vi "ConfigFlattenMicroscopeToXML.vi"(8 "error in (no error)":errorcluster, 11 "MicroscopeArray":string[][](array[string])) -> (0 "error out":errorcluster, 3 "MicrosocopeXML":string)   [LabVIEW 2018, in "Config.lvlib"]
uses:
  Config.lvlib
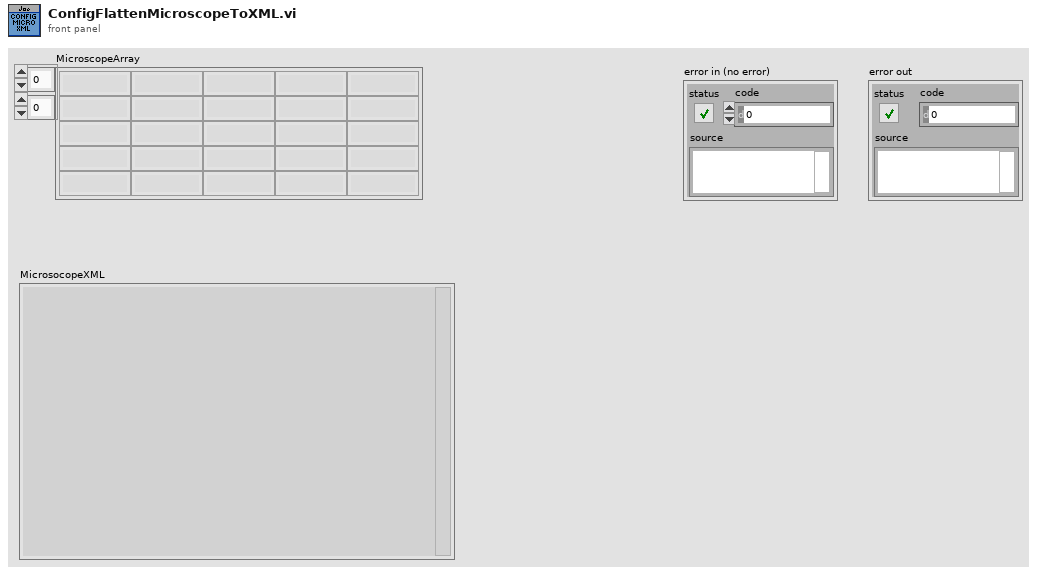
[diagram p1: front panel]
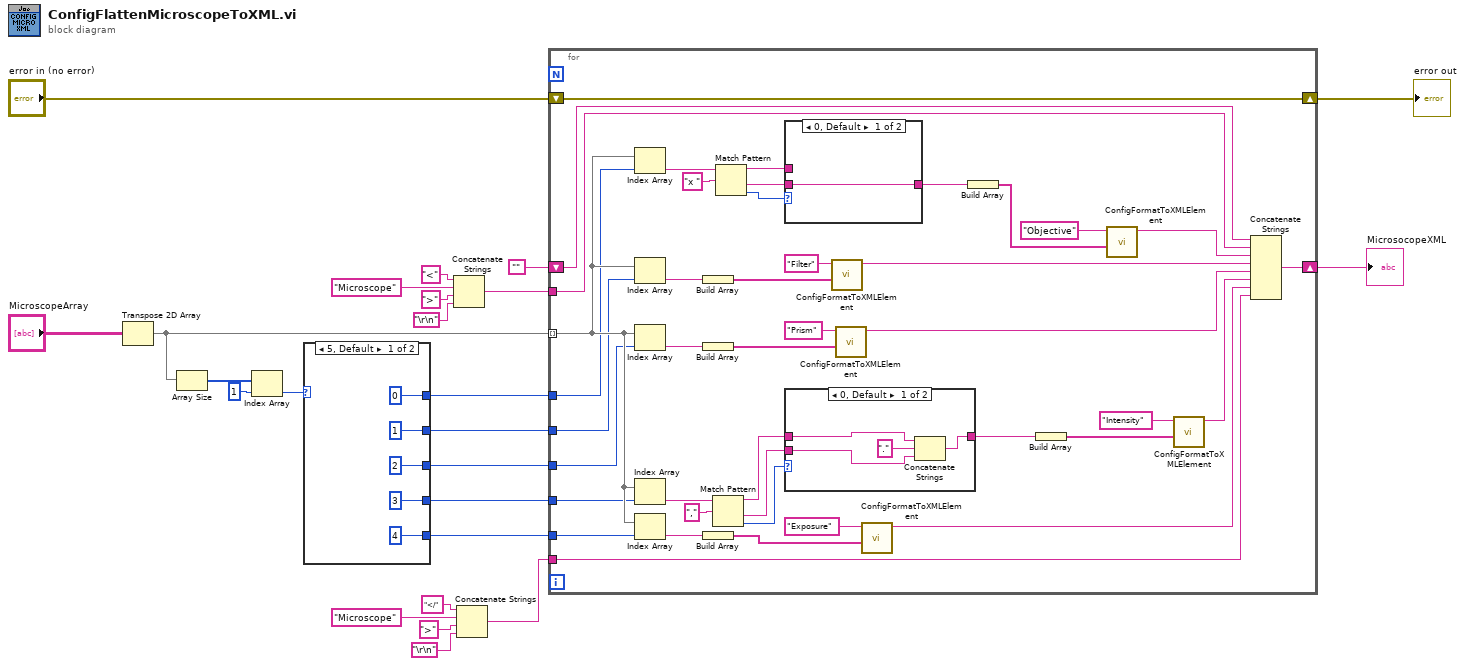
[diagram p0: block diagram]
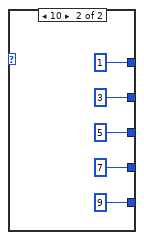
[diagram p2: hidden frame]
diagram:
  n1 = Transpose 2D Array(2D array="MicroscopeArray") -> (transposed array=w4:string[][])
  n2 = Array Size(array=w4) -> (size(s)=w3:i32[])
  n3 = Index Array(array=w3, index=1) -> (element=w1:i32)
  n4 = case shown="5, Default" w1 {
    tunnel: [0 ("index (row)") 1 ("index (row)")] -> w10
    tunnel: [1 ("index (row)") 3 ("index (row)")] -> w9
    tunnel: [2 ("index (row)") 5 ("index (row)")] -> w8
    tunnel: [3 ("index (row)") 7 ("index (row)")] -> w7
    tunnel: [4 ("index (row)") 9 ("index (row)")] -> w6
    frame 5, Default {
    }
    frame 10 {
    }
  }
  n5 = Concatenate Strings("<" ("string"), "Microscope" ("string"), ">" ("string"), "\r\n") -> (w13:string)
  n6 = Concatenate Strings("</" ("string"), "Microscope" ("string"), ">" ("string"), "\r\n") -> (w12:string)
  n7 = for {
    tunnel: w4 -> [w70] mode=indexing
    shift-right: [w71] -> w11
    shift-left: "" -> [w72]
    shift-right: [w75] -> w23
    shift-left: "error in (no error)" -> [w75]
    tunnel: w13 -> [w74]
    tunnel: w12 -> [w73]
    tunnel: w10 -> [w51]
    tunnel: w9 -> [w50]
    tunnel: w8 -> [w49]
    tunnel: w7 -> [w48]
    tunnel: w6 -> [w47]
    n8 = Index Array(array=w70, index=w51) -> (element=w46:string)
    n9 = Index Array(array=w70, index=w50) -> (element=w64:string)
    n10 = Index Array(array=w70, index=w49) -> (element=w61:string)
    n11 = Index Array(array=w70, index=w48) -> (element=w39:string)
    n12 = Index Array(array=w70, index=w47) -> (element=w58:string)
    n13 = Build Array(w64) -> (w65:string[])
    n14 = Build Array(w61) -> (w68:string[])
    n15 = Build Array(w58) -> (w66:string[])
    n16 = Match Pattern(string=w39, regular expression=",") -> (before substring=w38:string, after substring=w36:string, offset past match=w35:i32)  [unwired: 1 in, 1 out]
    n17 = Match Pattern(string=w46, regular expression="x ") -> (before substring=w43:string, after substring=w42:string, offset past match=w44:i32)  [unwired: 1 in, 1 out]
    n18 = case shown="0, Default" w44 {
      tunnel: [w81 w82] -> w45
      tunnel: w43 -> [_ w82]
      tunnel: w42 -> [w81 _]
      frame 0, Default {
      }
      frame -1 {
      }
    }
    n19 = case shown="0, Default" w35 {
      tunnel: [w78 w80] -> w37
      tunnel: w38 -> [w79 w80]
      tunnel: w36 -> [w76 _]
      frame 0, Default {
        n20 = Concatenate Strings(w79, "." ("string"), w76) -> (w78:string)
      }
      frame -1 {
      }
    }
    n21 = call "ConfigFormatToXMLElement.vi"("Value"=w65, "outer Tag"="Filter") -> ("Resulting String"=w55:string)  [unwired: 9 in]
    n22 = call "ConfigFormatToXMLElement.vi"("Value"=w68, "outer Tag"="Prism") -> ("Resulting String"=w54:string)  [unwired: 9 in]
    n23 = call "ConfigFormatToXMLElement.vi"("Value"=w66, "outer Tag"="Exposure") -> ("Resulting String"=w52:string)  [unwired: 9 in]
    n24 = Build Array(w45) -> (w69:string[])
    n25 = Build Array(w37) -> (w67:string[])
    n26 = call "ConfigFormatToXMLElement.vi"("Value"=w69, "outer Tag"="Objective") -> ("Resulting String"=w56:string)  [unwired: 9 in]
    n27 = call "ConfigFormatToXMLElement.vi"("Value"=w67, "outer Tag"="Intensity") -> ("Resulting String"=w53:string)  [unwired: 9 in]
    n28 = Concatenate Strings(w72, w74, w56, w55, w54, w53, w52, w73) -> (w71:string)
  }
  "error out" <- w23
  "MicrosocopeXML" <- w11
